vi "_Server Global.vi"() -> ()   [LabVIEW 2015]
uses:
  Type/_Brief Status.ctl
  Type/_Source Type.ctl
  Type/_Server Command.ctl
panel:
  out "CCLogicRef":refnum<vi>
  out "MethodPath":path
  in  "Plate #":u16=1
  out "APPI":bool
  out "BusyRef":refnum<vi>
  out "ReadyRef":refnum<vi>
  out "ErrorRef":refnum<vi>
  out "DataRef":refnum<vi>
  out "MessageRef":refnum<vi>
  out "LockedRef":refnum<vi>
  out "Data Queue":i32
  out "GetStatusRef":refnum<vi>
  out "CommandRef":refnum<vi>
  out "MSStatus":T1 {"Corona Discharge:" format="%#.2g"; "Vac. Pressure:" format="%#.2g"; "Nebulizer Gas 2:" format="%#.2g"; "Source 2 Type:" items=["None", "ESI", "APCI", "APPI", "MicroSpray"]; "Source 1 Type:" items=["None", "ESI", "APCI", "APPI", "MicroSpray"]}
  in  "# of Injections":u16=1 min=1 max=100 step=1
  in  "Inj Volume":dbl=10.0
  in  "Vial #":u16=1
  in  "Rack Type":u16=65
  out "PrepareMethod":bool
  out "Sim Run Time (mS)":u32
  out "Remaining Scans":i32
  # "For Manual LC Control"
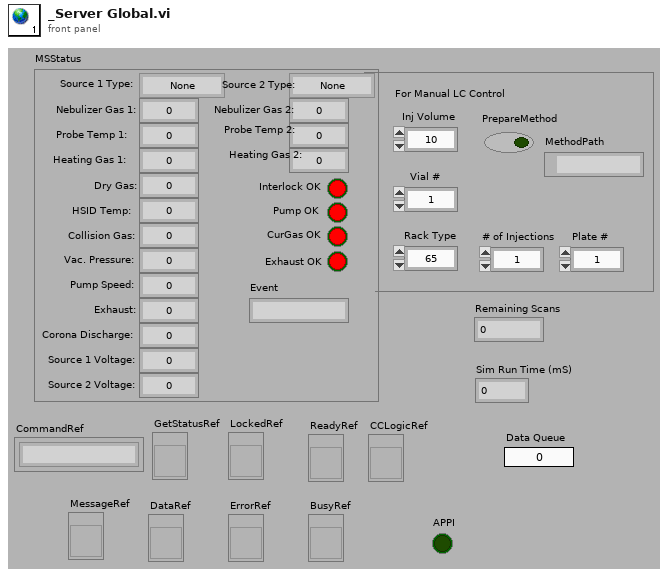
[diagram p1: front panel]
types:
  T1 = typedef "_Brief Status.ctl" = cluster{"Source 1 Type: ":T2, "Nebulizer Gas 1:":sgl, "Probe Temp 1: ":sgl, "Heating Gas 1:":sgl, "Source 2 Type:  ":T2, "Nebulizer Gas 2:":sgl, "Probe Temp 2: ":sgl, "Heating Gas 2:":sgl, "Dry Gas:":sgl, "HSID Temp:  ":sgl, "Collision Gas:":sgl, "Vac. Pressure: ":sgl, "Pump Speed:":sgl, "Exhaust:":sgl, "Interlock OK":bool, "CurGas OK":bool, "Pump OK":bool, "Exhaust OK":bool, "Event":string, "Corona Discharge:":sgl, "Source 1 Voltage:":sgl, "Source 2 Voltage:":sgl}
  T2 = typedef "_Source Type.ctl" = i8
diagram:
